vi "1.-Generador de Funciones en LabView con Ruido.vi"() -> ()   [LabVIEW 2020]
uses:
  <vilib>/measure/maspectr.llb/FFT Power Spectrum and PSD for 1 Chan.vi
  <vilib>/measure/NI_MAPro.lvlib
panel:
  out "error out":errorcluster
  in  "error in (no error)":errorcluster
  out "Waveform Graph 2":cluster{"f0":dbl, "df":dbl, "magnitude":dbl[]}(graph)
  out "Waveform Chart 2":dynamicdata(graph)
  in  "Frequency":dbl(knob)=60.0 scale=0.0..550.0
  out "Waveform Graph":cluster{"f0":dbl, "df":dbl, "magnitude":dbl[]}(graph)
  in  "stop":bool
  out "Waveform Chart":dynamicdata(graph)
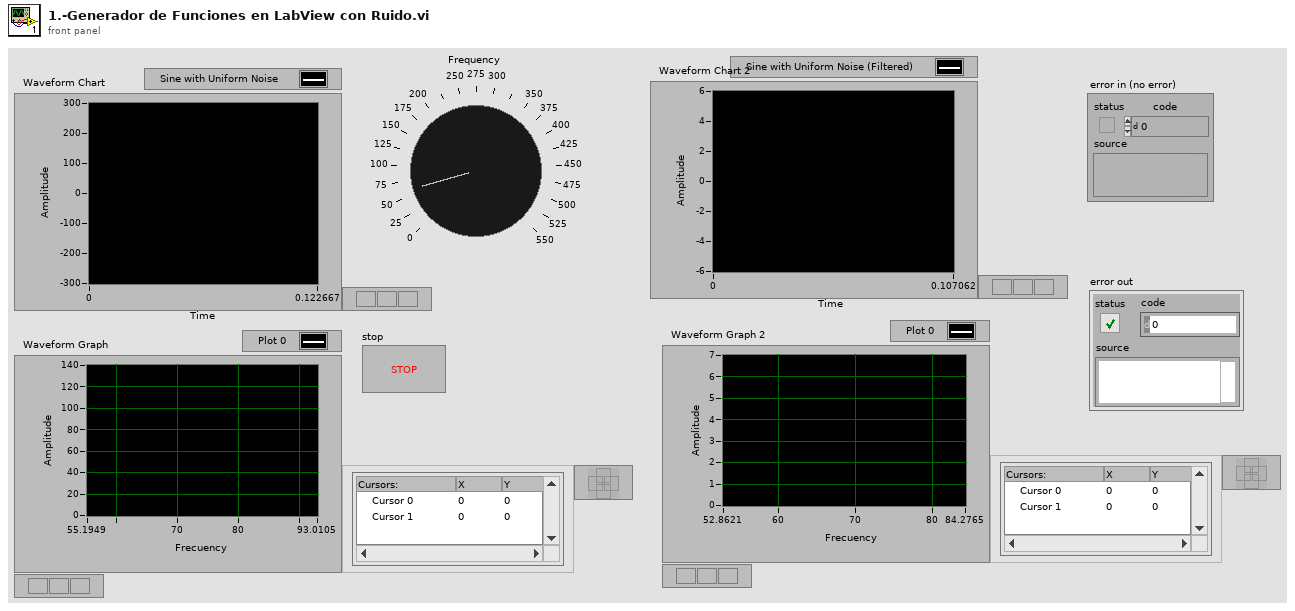
[diagram p1: front panel]
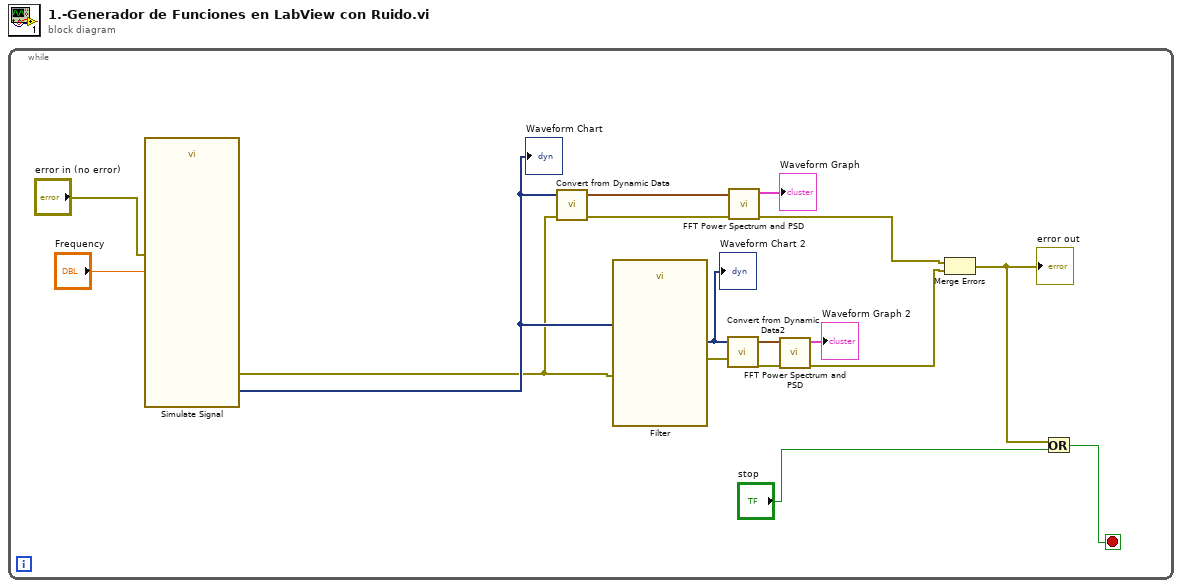
[diagram p0: block diagram]
diagram:
  n1 = while {
    stop <- w1 stop-if-true
    n2 = call "Simulate Signal"("Frequency"="Frequency", "error in (no error)"="error in (no error)") -> ("Sine with Uniform Noise"=w12:dynamicdata, "error out"=w7:errorcluster)  [unwired: 12 in]
    "Waveform Chart" <- w12
    n3 = call "Convert from Dynamic Data"("Dynamic Data Type"=w12) -> ("Waveform"=w15:waveform(dbl))  [unwired: 3 in]
    n4 = call "Filter"("error in (no error)"=w7, "Signal"=w12) -> ("error out"=w6:errorcluster, "Filtered Signal"=w9:dynamicdata)  [unwired: 8 in]
    "Waveform Chart 2" <- w9
    n5 = call "Convert from Dynamic Data2"("Dynamic Data Type"=w9) -> ("Waveform"=w10:waveform(dbl))  [unwired: 3 in]
    n6 = call-poly <vilib>:"FFT Power Spectrum and PSD.vi"("error in (no error)"=w7, "time signal"=w15) -> ("error out"=w5:errorcluster, "Power Spectrum / PSD"=→"Waveform Graph":cluster{"f0":dbl, "df":dbl, "magnitude":dbl[]})  [unwired: 6 in, 2 out]
    n7 = call-poly <vilib>:"FFT Power Spectrum and PSD.vi"("error in (no error)"=w6, "time signal"=w10) -> ("error out"=w4:errorcluster, "Power Spectrum / PSD"=→"Waveform Graph 2":cluster{"f0":dbl, "df":dbl, "magnitude":dbl[]})  [unwired: 6 in, 2 out]
    n8 = Merge Errors(w5, w4) -> (w2:errorcluster)
    "error out" <- w2
    n9 = Or(x=w2, y="stop") -> (x .or. y?=w1:bool)
  }
